vi "Enumeration.vi"() -> (3 "Enumeration":T1(c390))   [LabVIEW 2025, in "Config Library.lvlib" / "Read Config File.lvclass"]
uses:
  Read Config File.lvclass
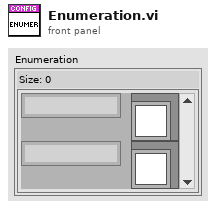
[diagram p1: front panel]
types:
  T1 = map{string, refnum<class "Read Config File.lvclass">}
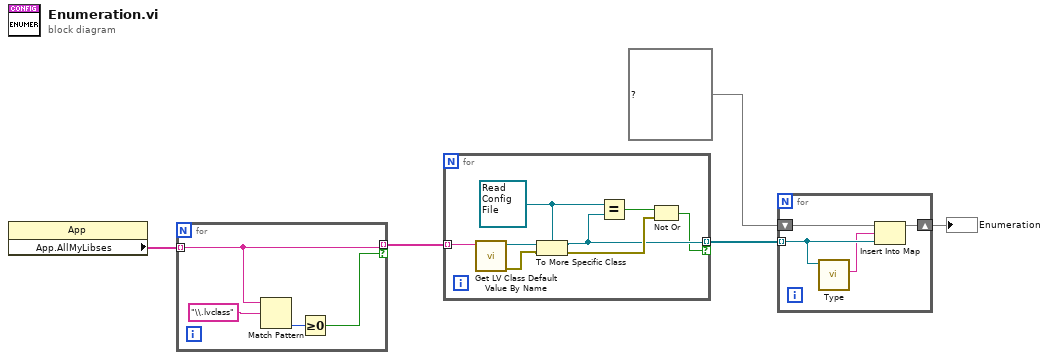
[diagram p0: block diagram]
diagram:
  n1 = property class="App"() -> ("App.AllMyLibses"=w5:string[])  [unwired: 2 in, 2 out]
  n2 = for {
    tunnel: w5 -> [w9] mode=indexing
    tunnel: [w9] -> w4 mode=indexing if=w7
    n3 = Match Pattern(string=w9, regular expression="\\.lvclass") -> (offset past match=w8:i32)  [unwired: 1 in, 3 out]
    n4 = Greater Or Equal To 0?(x=w8) -> (x >= 0?=w7:bool)
  }
  n5 = for {
    tunnel: w4 -> [w17] mode=indexing
    tunnel: [w11] -> w3 mode=indexing if=w10
    w14 = refnum<class "Read Config File.lvclass"> refnum ("Config Library.lvlib:Read Config File")
    n6 = call <vilib>:"Get LV Class Default Value By Name.vi"("class name"=w17) -> ("error out"=w15:errorcluster, "object"=w16:refnum<class>)  [unwired: 9 in]
    n7 = To More Specific Class(target class=w14, reference=w16, error in=w15) -> (specific class reference=w11:refnum<class "Read Config File.lvclass">, error out=w12:errorcluster)
    n8 = Equal?(x=w14, y=w11) -> (x = y?=w13:bool)
    n9 = Not Or(1:w12, 2:w13) -> (0:w10:bool)
  }
  n10 = for {
    tunnel: w3 -> [w19] mode=indexing
    shift-right: [w20] -> w1
    shift-left: T1 {} ("Map") -> [w21]
    n11 = call-dynamic "Type.vi"("Read Config File in"=w19) -> ("Name"=w18:string)  [unwired: 10 in]
    n12 = Insert Into Map(map in=w21, key=w18, value=w19) -> (map out=w20:T1)  [unwired: 2 out]
  }
  "Enumeration" <- w1
